vi "Construct_Optimal_Subtrack_(11-111)-2.vi"(6 "[IN] Indexes for Jumps":i32[](array[numeric]), 8 "error IN":errorcluster, 9 "[IN] Index of recon\nstructed tracks":i32, 10 "[IN] Clusters for Re\nconstructed Tracks":T1, 11 "[IN] Still connected\ntracks in group":T2) -> (0 "error OUT":errorcluster, 2 "[OUT] Clusters for Re\nconstructed Tracks":T1)   [LabVIEW 2013]
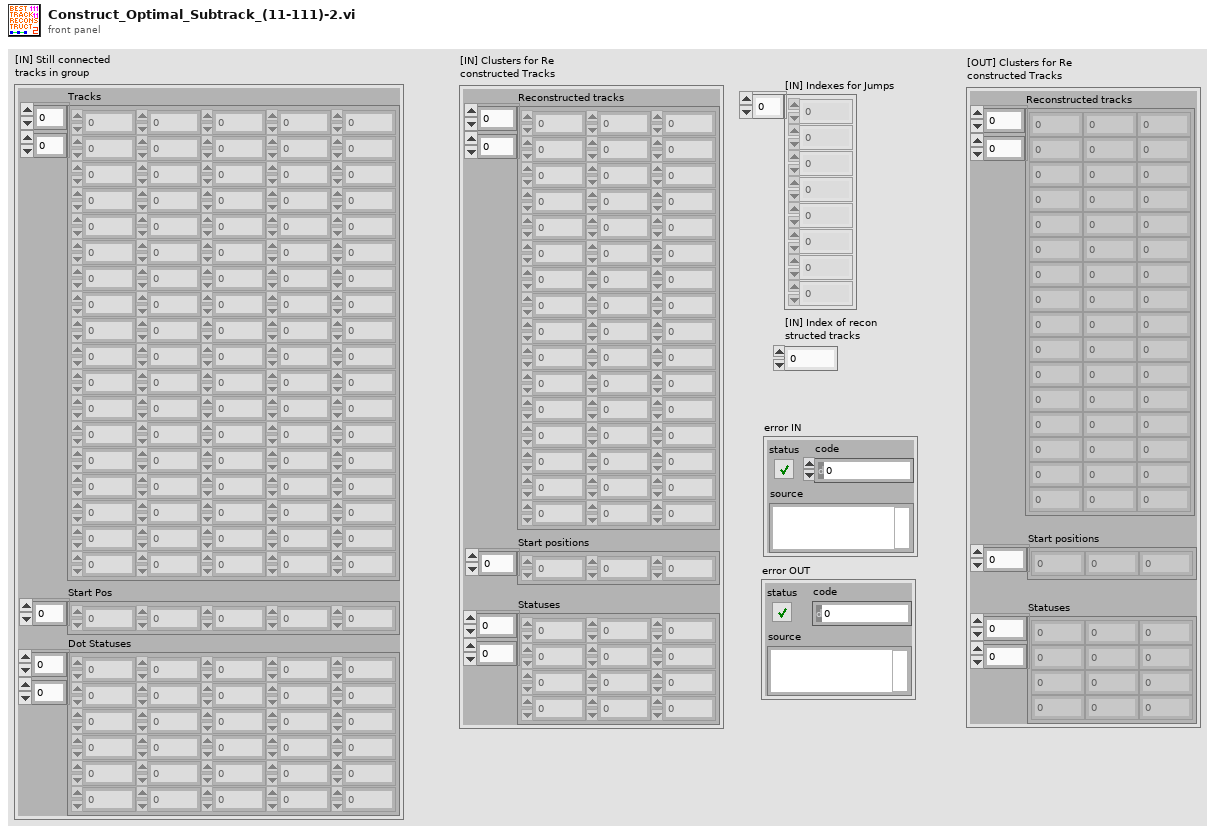
[diagram p1: front panel]
types:
  T1 = cluster{"Reconstructed tracks":dbl[][], "Start positions":i32[], "Statuses":i16[][]}
  T2 = cluster{"Tracks":dbl[][], "Start Pos":i32[], "Dot Statuses":i16[][]}
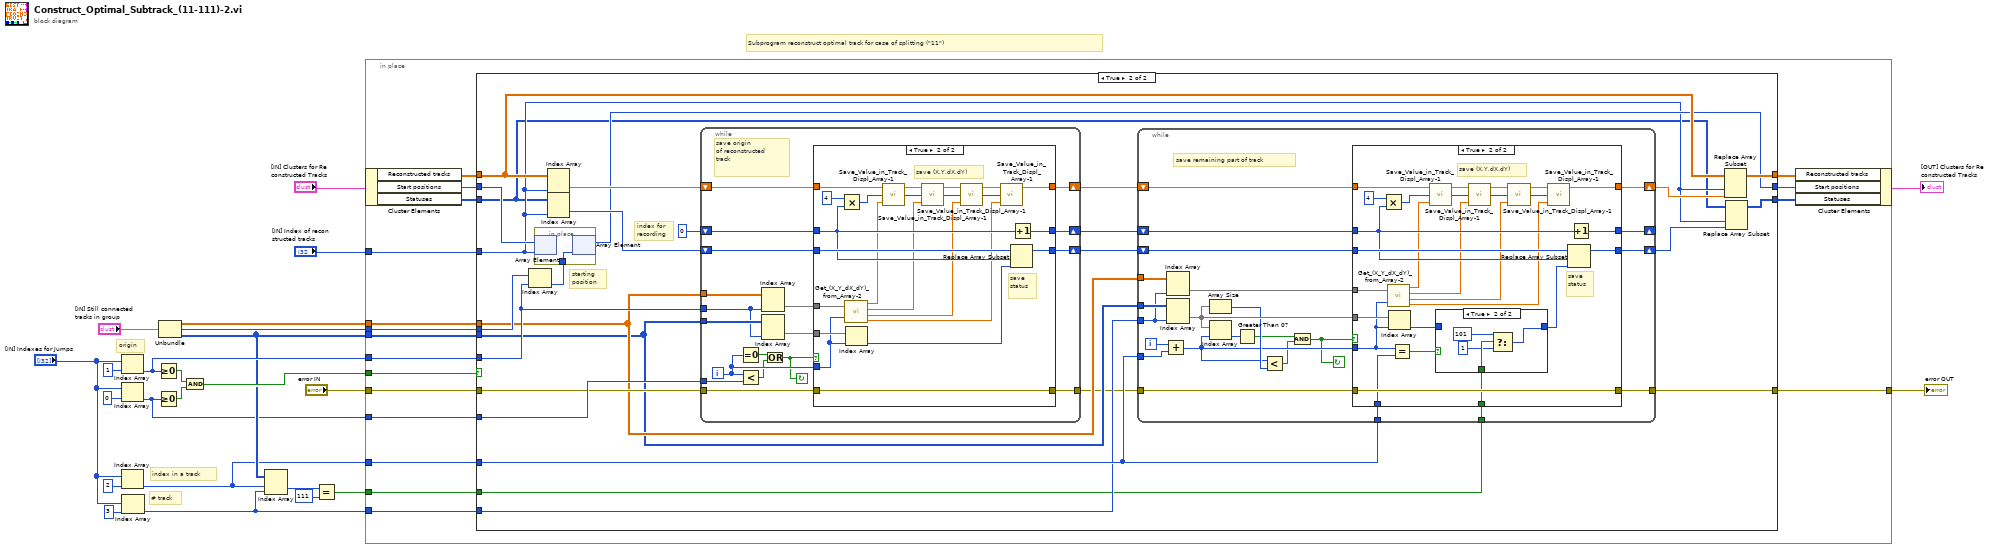
[diagram p0: block diagram]
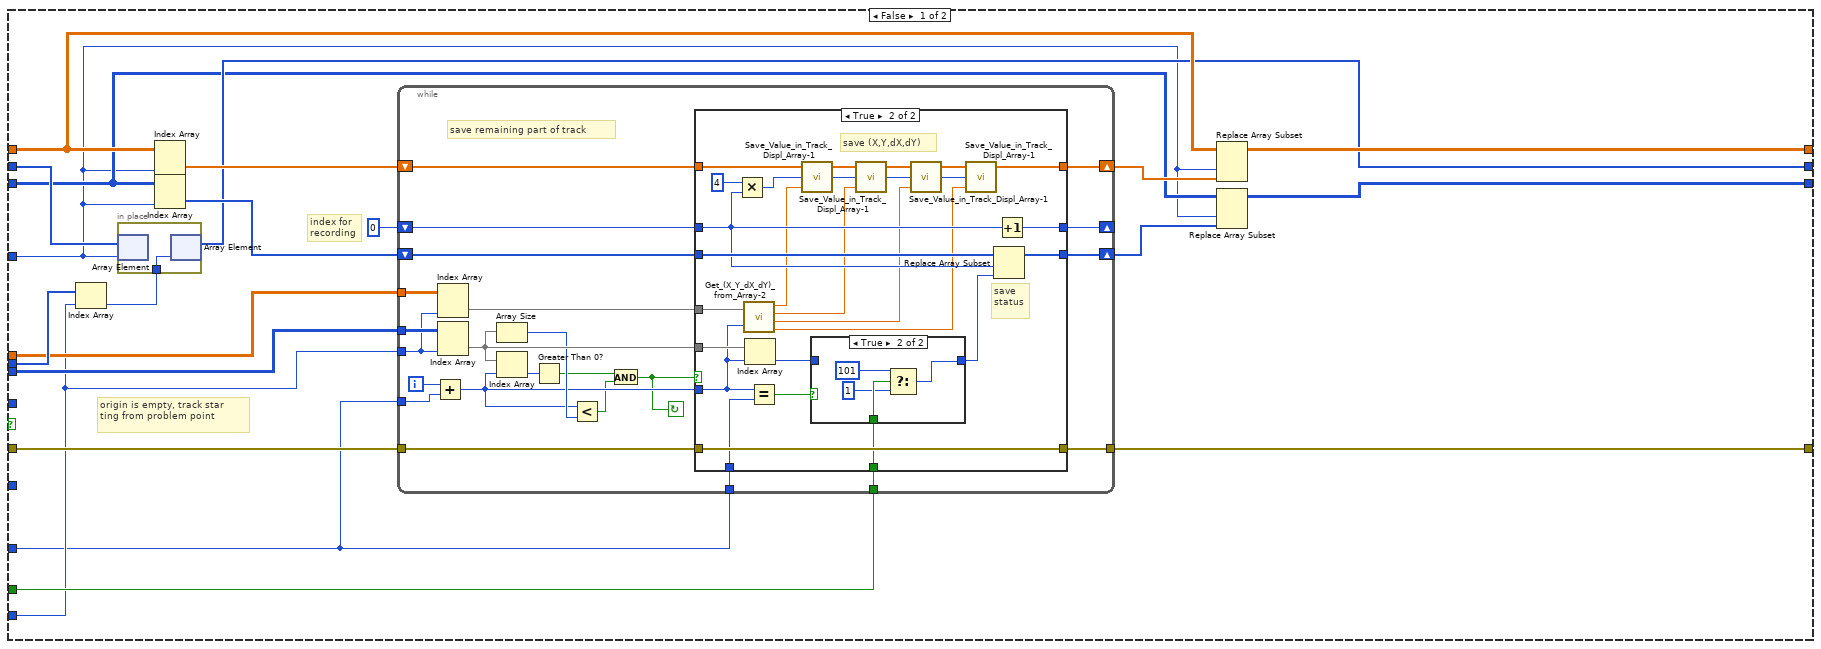
[diagram p2: hidden frame]
diagram:
  # "index in a track"
  # "# track"
  # "origin"
  # "Subprogram reconstruct optimal track for case of splitting (\"11\")"
  n1 = Index Array(array="[IN] Indexes for Jumps", index=1) -> (element=w11:i32)
  n2 = Index Array(array="[IN] Indexes for Jumps", index=0) -> (element=w7:i32)
  n3 = Index Array(array="[IN] Indexes for Jumps", index=2) -> (element=w5:i32)
  n4 = Index Array(array="[IN] Indexes for Jumps", index=3) -> (element=w4:i32)
  n5 = Greater Or Equal To 0?(x=w11) -> (x >= 0?=w15:bool)
  n6 = Greater Or Equal To 0?(x=w7) -> (x >= 0?=w14:bool)
  n7 = Unbundle("[IN] Still connected\ntracks in group") -> ("Tracks"=w8:dbl[][], "Start Pos"=w9:i32[], "Dot Statuses"=w10:i16[][])
  n8 = And(x=w15, y=w14) -> (x .and. y?=w13:bool)
  n9 = Index Array(array=w10, index (row)=w5, index (col)=w4) -> (element=w18:i16)
  n10 = Equal?(x=w18, y=i16 111) -> (x = y?=w3:bool)
  n11 = in-place {
    in-place-border: w13 -> [w42]
    in-place-border: "[IN] Index of recon\nstructed tracks" -> [w34]
    in-place-border: w11 -> [w41]
    in-place-border: w10 -> [w40]
    in-place-border: w9 -> [w39]
    in-place-border: w8 -> [w38]
    in-place-border: w7 -> [w33]
    in-place-border: "error IN" -> [w32]
    in-place-border: w5 -> [w31]
    in-place-border: w4 -> [w30]
    in-place-border: w3 -> [w29]
    in-place-border: [w25] -> w1
    n12 = in-place-cluster #1("[IN] Clusters for Re\nconstructed Tracks") -> ("Reconstructed tracks"=w35:dbl[][], "Start positions"=w37:i32[], "Statuses"=w36:i16[][])
    n13 = case shown="True" w42 {
      tunnel: w41 -> [_ w144]
      tunnel: w40 -> [w56 w136]
      tunnel: w39 -> [w63 w149]
      tunnel: w38 -> [w58 w138]
      tunnel: w37 -> [w61 w150]
      tunnel: w36 -> [w46 w126]
      tunnel: w35 -> [w51 w132]
      tunnel: w34 -> [w45 w128]
      tunnel: w33 -> [_ w143]
      tunnel: w32 -> [w54 w142]
      tunnel: w31 -> [w52 w137]
      tunnel: w30 -> [w53 w135]
      tunnel: w29 -> [w55 w133]
      tunnel: [w50 w130] -> w28
      tunnel: [w48 w129] -> w27
      tunnel: [w43 w125] -> w26
      tunnel: [w47 w124] -> w25
      frame False {
        # "index for\nrecording"
        # "origin is empty, track star\nting from problem point"
        n14 = Index Array(array=w63, index=w53) -> (element=w62:i32)
        n15 = in-place {
          in-place-border: w62 -> [w64]
          n16 = in-place-array #2(w61, w45) -> ()  [unwired: 1 out]
          n17 = in-place-array #2(w64) -> (w48:i32[])  [unwired: 1 out]
        }
        n18 = Index Array(array=w51, index (col)=w45) -> (element=w60:dbl[])  [unwired: 1 in]
        n19 = Index Array(array=w46, index (col)=w45) -> (element=w57:i16[])  [unwired: 1 in]
        n20 = while {
          tunnel: w58 -> [w87]
          tunnel: w56 -> [w86]
          tunnel: w53 -> [w85]
          shift-right: [w80] -> w49
          shift-left: w60 -> [w84]
          shift-right: [w78] -> w44
          shift-left: w57 -> [w82]
          shift-right: [w79] -> _
          shift-left: 0 -> [w81]
          tunnel: w52 -> [w76]
          tunnel: w54 -> [w68]
          tunnel: [w67] -> w47
          tunnel: w52 -> [w66]
          tunnel: w55 -> [w65]
          i -> [w77]
          stop <- w69 continue-if-true
          # "save remaining part of track"
          n21 = Add(x=w77, y=w76) -> (x+y=w72:i32)
          n22 = Index Array(array=w87, index (col)=w85) -> (element=w83:dbl[])  [unwired: 1 in]
          n23 = Index Array(array=w86, index (col)=w85) -> (element=w75:i16[])  [unwired: 1 in]
          n24 = Array Size(array=w75) -> (size(s)=w73:i32)
          n25 = Index Array(array=w75, index=w72) -> (element=w74:i16)
          n26 = Greater Than 0?(x=w74) -> (x > 0?=w71:bool)
          n27 = Less?(x=w72, y=w73) -> (x < y?=w70:bool)
          n28 = And(x=w71, y=w70) -> (x .and. y?=w69:bool)
          n29 = case shown="True" w69 {
            tunnel: w84 -> [w91 w104]
            tunnel: w83 -> [_ w118]
            tunnel: w75 -> [_ w117]
            tunnel: w72 -> [_ w110]
            tunnel: w82 -> [w89 w115]
            tunnel: [w89 w114] -> w78
            tunnel: [w91 w92] -> w80
            tunnel: w81 -> [w90 w113]
            tunnel: [w90 w112] -> w79
            tunnel: w68 -> [w88 w111]
            tunnel: [w88 w111] -> w67
            tunnel: w66 -> [_ w109]
            tunnel: w65 -> [_ w105]
            frame False {
            }
            frame True {
              # "save (X,Y,dX,dY)"
              # "save\nstatus"
              n30 = Multiply(x=4, y=w113) -> (x*y=w103:i32)
              n31 = call "Get_(X_Y_dX_dY)_from_Array-2.vi"("(X,Y,dX,dY)"=w118, "Index of Displacement"=w110) -> ("X"=w102:dbl, "Y"=w99:dbl, "dX"=w97:dbl, "dY"=w93:dbl)
              n32 = Index Array(array=w117, index=w110) -> (element=w107:i16)
              n33 = Equal?(x=w110, y=w109) -> (x = y?=w108:bool)
              n34 = call "Save_Value_in_Track_Displ_Array-1.vi"("[IN] Value"=w102, "[IN] Index"=w103, "[IN] Empty tracks\nfor points saving"=w104) -> ("[OUT] Index ++"=w100:i32, "[OUT Track with saved value"=w101:dbl[])  [unwired: 1 in]
              n35 = case shown="True" w108 {
                tunnel: w107 -> [w119 _]
                tunnel: [w119 w120] -> w106
                tunnel: w105 -> [_ w123]
                frame False {
                }
                frame True {
                  n36 = Select(t=i16 101 ("element"), s=w123, f=i16 1 ("element")) -> (s? t:f=w120:i16)
                }
              }
              n37 = call "Save_Value_in_Track_Displ_Array-1.vi"("[IN] Value"=w99, "[IN] Index"=w100, "[IN] Empty tracks\nfor points saving"=w101) -> ("[OUT] Index ++"=w96:i32, "[OUT Track with saved value"=w98:dbl[])  [unwired: 1 in]
              n38 = call "Save_Value_in_Track_Displ_Array-1.vi"("[IN] Value"=w97, "[IN] Index"=w96, "[IN] Empty tracks\nfor points saving"=w98) -> ("[OUT] Index ++"=w94:i32, "[OUT Track with saved value"=w95:dbl[])  [unwired: 1 in]
              n39 = call "Save_Value_in_Track_Displ_Array-1.vi"("[IN] Value"=w93, "[IN] Index"=w94, "[IN] Empty tracks\nfor points saving"=w95) -> ("[OUT Track with saved value"=w92:dbl[])  [unwired: 1 in, 1 out]
              n40 = Replace Array Subset(array=w115, new element=w106, index=w113) -> (w114:i16[])
              n41 = Increment(x=w113) -> (x+1=w112:i32)
            }
          }
        }
        n42 = Replace Array Subset(array=w51, new element=w49, index (col)=w45) -> (w50:dbl[][])  [unwired: 1 in]
        n43 = Replace Array Subset(array=w46, new element=w44, index (col)=w45) -> (w43:i16[][])  [unwired: 1 in]
      }
      frame True {
        # "index for\nrecording"
        # "starting\nposition"
        n44 = Index Array(array=w149, index=w144) -> (element=w148:i32)
        n45 = in-place {
          in-place-border: w148 -> [w255]
          n46 = in-place-array #3(w150, w128) -> ()  [unwired: 1 out]
          n47 = in-place-array #3(w255) -> (w129:i32[])  [unwired: 1 out]
        }
        n48 = Index Array(array=w132, index (col)=w128) -> (element=w146:dbl[])  [unwired: 1 in]
        n49 = Index Array(array=w126, index (col)=w128) -> (element=w145:i16[])  [unwired: 1 in]
        n50 = while {
          tunnel: w143 -> [w224]
          tunnel: w138 -> [w227]
          tunnel: w136 -> [w226]
          tunnel: w144 -> [w225]
          shift-right: [w218] -> w141
          shift-left: w146 -> [w223]
          shift-right: [w216] -> w139
          shift-left: w145 -> [w220]
          shift-right: [w217] -> w140
          shift-left: 0 -> [w219]
          tunnel: w142 -> [w215]
          tunnel: [w214] -> w134
          i -> [w213]
          stop <- w210 continue-if-true
          # "save origin \nof reconstructed \ntrack"
          n51 = Equal To 0?(x=w213) -> (x = 0?=w212:bool)
          n52 = Less?(x=w213, y=w224) -> (x < y?=w211:bool)
          n53 = Index Array(array=w227, index (col)=w225) -> (element=w222:dbl[])  [unwired: 1 in]
          n54 = Index Array(array=w226, index (col)=w225) -> (element=w221:i16[])  [unwired: 1 in]
          n55 = Or(x=w212, y=w211) -> (x .or. y?=w210:bool)
          n56 = case shown="True" w210 {
            tunnel: w223 -> [w231 w244]
            tunnel: w222 -> [_ w254]
            tunnel: w221 -> [_ w253]
            tunnel: w213 -> [_ w249]
            tunnel: w220 -> [w229 w251]
            tunnel: [w229 w248] -> w216
            tunnel: [w231 w233] -> w218
            tunnel: w219 -> [w230 w247]
            tunnel: [w230 w246] -> w217
            tunnel: w215 -> [w228 w245]
            tunnel: [w228 w245] -> w214
            frame False {
            }
            frame True {
              # "save (X,Y,dX,dY)"
              # "save\nstatus"
              n57 = Multiply(x=4, y=w247) -> (x*y=w242:i32)
              n58 = call "Get_(X_Y_dX_dY)_from_Array-2.vi"("(X,Y,dX,dY)"=w254, "Index of Displacement"=w249) -> ("X"=w243:dbl, "Y"=w239:dbl, "dX"=w237:dbl, "dY"=w234:dbl)
              n59 = Index Array(array=w253, index=w249) -> (element=w250:i16)
              n60 = call "Save_Value_in_Track_Displ_Array-1.vi"("[IN] Value"=w243, "[IN] Index"=w242, "[IN] Empty tracks\nfor points saving"=w244) -> ("[OUT] Index ++"=w240:i32, "[OUT Track with saved value"=w241:dbl[])  [unwired: 1 in]
              n61 = call "Save_Value_in_Track_Displ_Array-1.vi"("[IN] Value"=w239, "[IN] Index"=w240, "[IN] Empty tracks\nfor points saving"=w241) -> ("[OUT] Index ++"=w236:i32, "[OUT Track with saved value"=w238:dbl[])  [unwired: 1 in]
              n62 = call "Save_Value_in_Track_Displ_Array-1.vi"("[IN] Value"=w237, "[IN] Index"=w236, "[IN] Empty tracks\nfor points saving"=w238) -> ("[OUT] Index ++"=w232:i32, "[OUT Track with saved value"=w235:dbl[])  [unwired: 1 in]
              n63 = call "Save_Value_in_Track_Displ_Array-1.vi"("[IN] Value"=w234, "[IN] Index"=w232, "[IN] Empty tracks\nfor points saving"=w235) -> ("[OUT Track with saved value"=w233:dbl[])  [unwired: 1 in, 1 out]
              n64 = Replace Array Subset(array=w251, new element=w250, index=w247) -> (w248:i16[])
              n65 = Increment(x=w247) -> (x+1=w246:i32)
            }
          }
        }
        n66 = while {
          tunnel: w138 -> [w173]
          tunnel: w136 -> [w172]
          tunnel: w135 -> [w171]
          shift-right: [w166] -> w131
          shift-left: w141 -> [w170]
          shift-right: [w164] -> w127
          shift-left: w139 -> [w168]
          shift-right: [w165] -> _
          shift-left: w140 -> [w167]
          tunnel: w137 -> [w162]
          tunnel: w134 -> [w154]
          tunnel: [w153] -> w124
          tunnel: w137 -> [w152]
          tunnel: w133 -> [w151]
          i -> [w163]
          stop <- w155 continue-if-true
          # "save remaining part of track"
          n67 = Add(x=w163, y=w162) -> (x+y=w158:i32)
          n68 = Index Array(array=w173, index (col)=w171) -> (element=w169:dbl[])  [unwired: 1 in]
          n69 = Index Array(array=w172, index (col)=w171) -> (element=w161:i16[])  [unwired: 1 in]
          n70 = Array Size(array=w161) -> (size(s)=w159:i32)
          n71 = Index Array(array=w161, index=w158) -> (element=w160:i16)
          n72 = Greater Than 0?(x=w160) -> (x > 0?=w157:bool)
          n73 = Less?(x=w158, y=w159) -> (x < y?=w156:bool)
          n74 = And(x=w157, y=w156) -> (x .and. y?=w155:bool)
          n75 = case shown="True" w155 {
            tunnel: w170 -> [w177 w190]
            tunnel: w169 -> [_ w204]
            tunnel: w161 -> [_ w203]
            tunnel: w158 -> [_ w196]
            tunnel: w168 -> [w175 w201]
            tunnel: [w175 w200] -> w164
            tunnel: [w177 w178] -> w166
            tunnel: w167 -> [w176 w199]
            tunnel: [w176 w198] -> w165
            tunnel: w154 -> [w174 w197]
            tunnel: [w174 w197] -> w153
            tunnel: w152 -> [_ w195]
            tunnel: w151 -> [_ w191]
            frame False {
            }
            frame True {
              # "save (X,Y,dX,dY)"
              # "save\nstatus"
              n76 = Multiply(x=4, y=w199) -> (x*y=w189:i32)
              n77 = call "Get_(X_Y_dX_dY)_from_Array-2.vi"("(X,Y,dX,dY)"=w204, "Index of Displacement"=w196) -> ("X"=w188:dbl, "Y"=w185:dbl, "dX"=w183:dbl, "dY"=w179:dbl)
              n78 = Index Array(array=w203, index=w196) -> (element=w193:i16)
              n79 = Equal?(x=w196, y=w195) -> (x = y?=w194:bool)
              n80 = call "Save_Value_in_Track_Displ_Array-1.vi"("[IN] Value"=w188, "[IN] Index"=w189, "[IN] Empty tracks\nfor points saving"=w190) -> ("[OUT] Index ++"=w186:i32, "[OUT Track with saved value"=w187:dbl[])  [unwired: 1 in]
              n81 = case shown="True" w194 {
                tunnel: w193 -> [w205 _]
                tunnel: [w205 w206] -> w192
                tunnel: w191 -> [_ w209]
                frame False {
                }
                frame True {
                  n82 = Select(t=i16 101 ("element"), s=w209, f=i16 1 ("element")) -> (s? t:f=w206:i16)
                }
              }
              n83 = call "Save_Value_in_Track_Displ_Array-1.vi"("[IN] Value"=w185, "[IN] Index"=w186, "[IN] Empty tracks\nfor points saving"=w187) -> ("[OUT] Index ++"=w182:i32, "[OUT Track with saved value"=w184:dbl[])  [unwired: 1 in]
              n84 = call "Save_Value_in_Track_Displ_Array-1.vi"("[IN] Value"=w183, "[IN] Index"=w182, "[IN] Empty tracks\nfor points saving"=w184) -> ("[OUT] Index ++"=w180:i32, "[OUT Track with saved value"=w181:dbl[])  [unwired: 1 in]
              n85 = call "Save_Value_in_Track_Displ_Array-1.vi"("[IN] Value"=w179, "[IN] Index"=w180, "[IN] Empty tracks\nfor points saving"=w181) -> ("[OUT Track with saved value"=w178:dbl[])  [unwired: 1 in, 1 out]
              n86 = Replace Array Subset(array=w201, new element=w192, index=w199) -> (w200:i16[])
              n87 = Increment(x=w199) -> (x+1=w198:i32)
            }
          }
        }
        n88 = Replace Array Subset(array=w132, new element=w131, index (col)=w128) -> (w130:dbl[][])  [unwired: 1 in]
        n89 = Replace Array Subset(array=w126, new element=w127, index (col)=w128) -> (w125:i16[][])  [unwired: 1 in]
      }
    }
    n90 = in-place-cluster #1("Reconstructed tracks"=w28, "Start positions"=w27, "Statuses"=w26) -> (→"[OUT] Clusters for Re\nconstructed Tracks":T1)
  }
  "error OUT" <- w1
